vi "Parse U8 Ctl Regs.vi"(9 "NTeeths In":T6, 10 "FullyCustomTeeths In":T4, 11 "U8":T2[](array[typedef])) -> (1 "NTeeths Out":T6, 2 "FullyCustomTeeths In":T4)   [LabVIEW 2011, in "Engine Sim System Explorer.lvlib"]
uses:
  Engine Sim System Explorer.lvlib
  TypeDefs/NTeethRegs.ctl
  TypeDefs/FullyCustomRegs.ctl
  <userlib>/_FPGA Interface Advanced Tools/FPGA Bitfile Utility/TypeDefs/Scalar Register.ctl
  <userlib>/_FPGA Interface Advanced Tools/FPGA Bitfile Utility/FPGA Bitfile Utility.lvlib
panel:
  in  "FullyCustomTeeths Profile Names":T1(array[cluster])
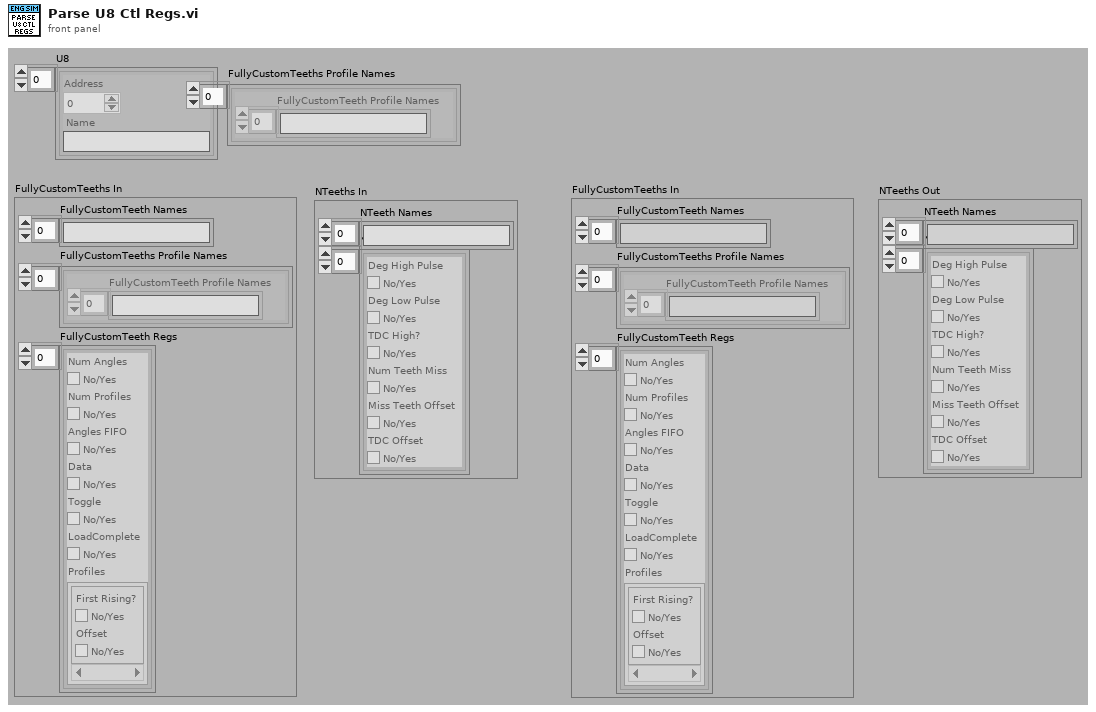
[diagram p1: front panel]
types:
  T1 = cluster{"FullyCustomTeeth Profile Names":string[]}[]
  T2 = typedef "FPGA Bitfile Utility.lvlib/Scalar Register.ctl" = cluster{"Address":u32, "Name":string}
  T3 = typedef "Engine Sim System Explorer.lvlib/FullyCustomRegs.ctl" = cluster{"Num Angles":bool, "Num Profiles":bool, "Angles FIFO":bool, "Data":bool, "Toggle":bool, "LoadComplete":bool, "Profiles":cluster{"First Rising?":bool, "Offset":bool}[]}
  T4 = cluster{"FullyCustomTeeth Names":string[], "FullyCustomTeeths Profile Names":cluster{"FullyCustomTeeth Profile Names":string[]}[], "FullyCustomTeeth Regs":T3[]}
  T5 = typedef "Engine Sim System Explorer.lvlib/NTeethRegs.ctl" = cluster{"Deg High Pulse":bool, "Deg Low Pulse":bool, "TDC High?":bool, "Num Teeth Miss":bool, "Miss Teeth Offset":bool, "TDC Offset":bool}
  T6 = cluster{"NTeeth Names":string[], "NTeeth Regs":T5[]}
  T7 = cluster{"FullyCustomTeeth Profile Names":string[]}
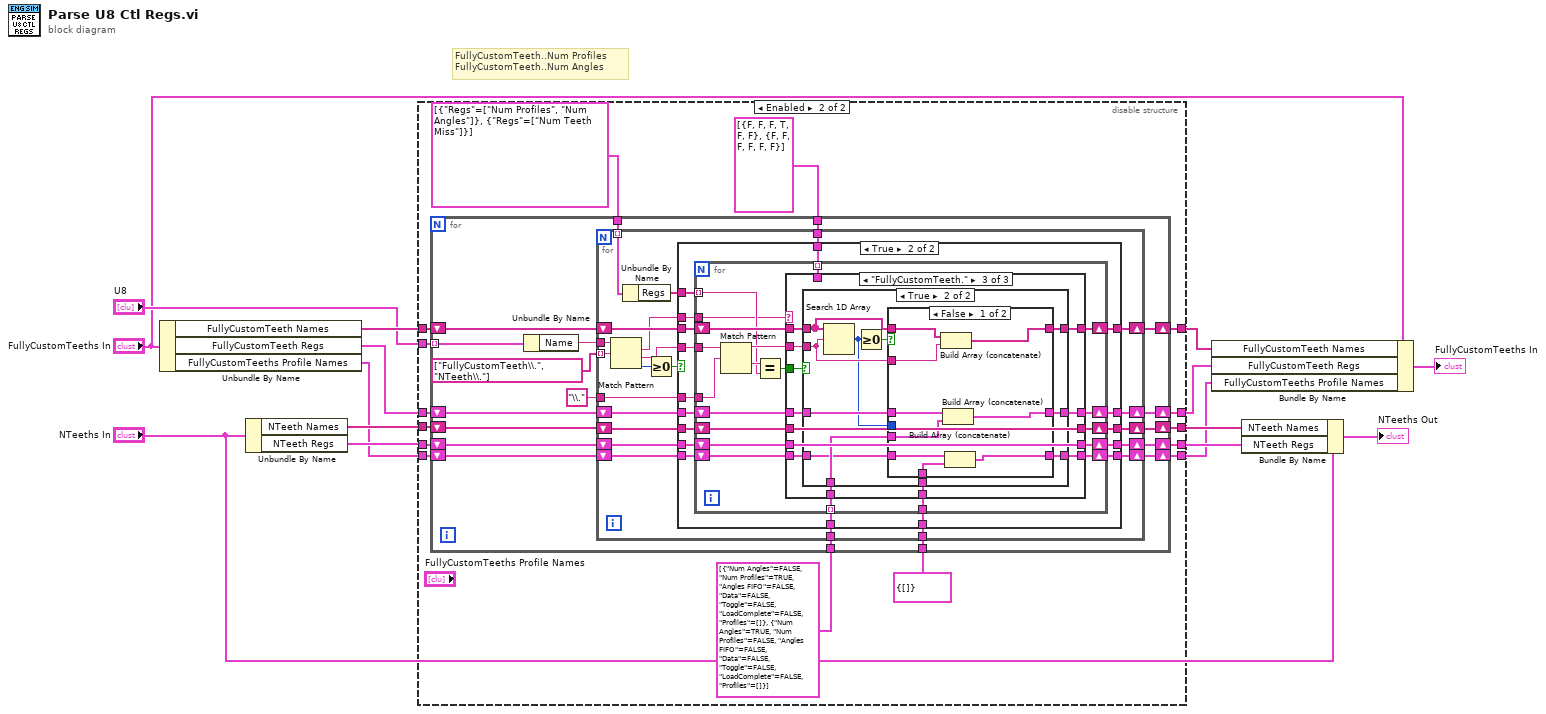
[diagram p0: block diagram]
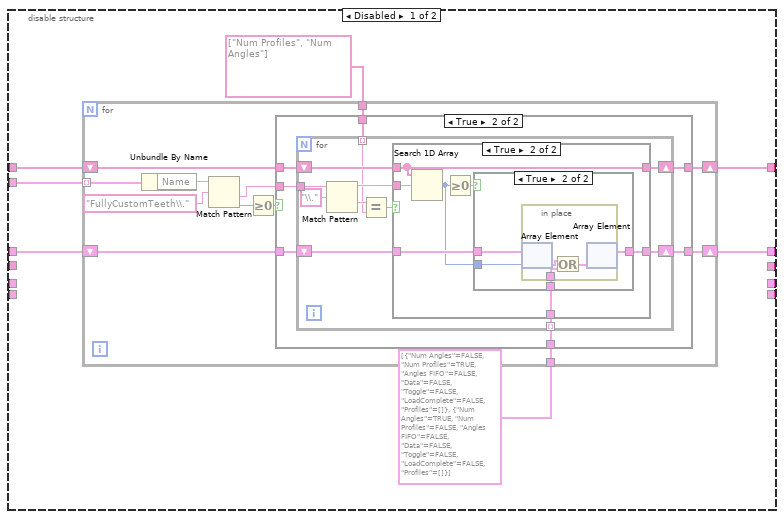
[diagram p2: hidden frame]
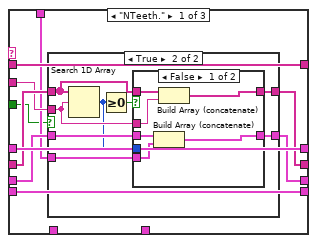
[diagram p7: hidden frame]
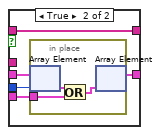
[diagram p9: hidden frame]
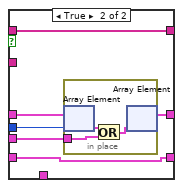
[diagram p12: hidden frame]
diagram:
  # "FullyCustomTeeth..Num Profiles\nFullyCustomTeeth..Num Angles"
  n1 = Unbundle By Name("FullyCustomTeeths In") -> ("FullyCustomTeeth Names"=w6:string[], "FullyCustomTeeth Regs"=w7:T3[], "FullyCustomTeeths Profile Names"=w2:T1)
  n2 = Unbundle By Name("NTeeths In") -> ("NTeeth Names"=w8:string[], "NTeeth Regs"=w9:T5[])
  n3 = disable-structure shown="Enabled" {
    disable-tunnel: w6 -> [w22 w85]
    disable-tunnel: w7 -> [w21 w84]
    disable-tunnel: "U8" -> [w20 w86]
    disable-tunnel: [w17 w83] -> w11
    disable-tunnel: [w16 w82] -> w10
    disable-tunnel: w9 -> [_ w79]
    disable-tunnel: w8 -> [_ w78]
    disable-tunnel: [_ w77] -> w14
    disable-tunnel: [_ w76] -> w15
    disable-tunnel: w2 -> [_ w75]
    disable-tunnel: [_ w73] -> w1
    frame Disabled {
      n4 = for {
        tunnel: w20 -> [w34] mode=indexing
        tunnel: T3[] [{"Num Angles"=FALSE, "Num Profiles"=TRUE, "Angles FIFO"=FALSE, "Data"=FALSE, "Toggle"=FALSE, "LoadComplete"=FALSE, "Profiles"=[]}, {"Num Angles"=TRUE, "Num Profiles"=FALSE, "Angles FIFO"=FALSE, "Data"=FALSE, "Toggle"=FALSE, "LoadComplete"=FALSE, "Profiles"=[]}] -> [w28]
        shift-right: [w27] -> w17
        shift-left: w21 -> [w26]
        shift-right: [w25] -> w16
        shift-left: w22 -> [w24]
        tunnel: string[] ["Num Profiles", "Num Angles"] ("Regs") -> [w23]
        n5 = Unbundle By Name(w34) -> ("Name"=w33:string)
        n6 = Match Pattern(string=w33, regular expression="FullyCustomTeeth\\.") -> (after substring=w29:string, offset past match=w31:i32)  [unwired: 1 in, 2 out]
        n7 = Greater Or Equal To 0?(x=w31) -> (x >= 0?=w30:bool)
        n8 = case shown="True" w30 {
          tunnel: w29 -> [_ w43]
          tunnel: w28 -> [_ w42]
          tunnel: [w35 w41] -> w27
          tunnel: w26 -> [w35 w40]
          tunnel: [w36 w39] -> w25
          tunnel: w24 -> [w36 w38]
          tunnel: w23 -> [_ w37]
          frame False {
          }
          frame True {
            n9 = for {
              tunnel: w43 -> [w54]
              tunnel: w42 -> [w49] mode=indexing
              tunnel: w37 -> [w44] mode=indexing
              shift-right: [w46] -> w39
              shift-left: w38 -> [w45]
              shift-right: [w48] -> w41
              shift-left: w40 -> [w47]
              n10 = Match Pattern(string=w54, regular expression="\\.") -> (before substring=w50:string, after substring=w52:string)  [unwired: 1 in, 2 out]
              n11 = Equal?(x=w52, y=w44) -> (x = y?=w51:bool)
              n12 = case shown="True" w51 {
                tunnel: w50 -> [_ w63]
                tunnel: w49 -> [_ w59]
                tunnel: [w55 w58] -> w48
                tunnel: w47 -> [w55 w60]
                tunnel: [w56 w62] -> w46
                tunnel: w45 -> [w56 w62]
                frame False {
                }
                frame True {
                  n13 = Search 1D Array(1D array=w62, element=w63) -> (index of element=w57:i32)  [unwired: 1 in]
                  n14 = Greater Or Equal To 0?(x=w57) -> (x >= 0?=w61:bool)
                  n15 = case shown="True" w61 {
                    tunnel: w60 -> [w64 w68]
                    tunnel: w59 -> [_ w67]
                    tunnel: [w64 w66] -> w58
                    tunnel: w57 -> [_ w65]
                    frame False {
                    }
                    frame True {
                      n16 = in-place {
                        in-place-border: w67 -> [w70]
                        n17 = in-place-array #1(w68, w65) -> (w71:T3)
                        n18 = Or(x=w71, y=w70) -> (x .or. y?=w69:T3)
                        n19 = in-place-array #1(w69) -> (w66:T3[])  [unwired: 1 out]
                      }
                    }
                  }
                }
              }
            }
          }
        }
      }
    }
    frame Enabled {
      n20 = for {
        tunnel: w86 -> [w104] mode=indexing
        tunnel: T3[] [{"Num Angles"=FALSE, "Num Profiles"=TRUE, "Angles FIFO"=FALSE, "Data"=FALSE, "Toggle"=FALSE, "LoadComplete"=FALSE, "Profiles"=[]}, {"Num Angles"=TRUE, "Num Profiles"=FALSE, "Angles FIFO"=FALSE, "Data"=FALSE, "Toggle"=FALSE, "LoadComplete"=FALSE, "Profiles"=[]}] -> [w102]
        shift-right: [w101] -> w83
        shift-left: w84 -> [w100]
        shift-right: [w99] -> w82
        shift-left: w85 -> [w98]
        tunnel: cluster{"Regs":string[]}[] [{"Regs"=["Num Profiles", "Num Angles"]}, {"Regs"=["Num Teeth Miss"]}] -> [w96]
        shift-right: [w95] -> w76
        shift-left: w79 -> [w94]
        tunnel: T5[] [{"Deg High Pulse"=FALSE, "Deg Low Pulse"=FALSE, "TDC High?"=FALSE, "Num Teeth Miss"=TRUE, "Miss Teeth Offset"=FALSE, "TDC Offset"=FALSE}, {"Deg High Pulse"=FALSE, "Deg Low Pulse"=FALSE, "TDC High?"=FALSE, "Num Teeth Miss"=FALSE, "Miss Teeth Offset"=FALSE, "TDC Offset"=FALSE}] -> [w93]
        shift-right: [w91] -> w77
        shift-left: w78 -> [w90]
        shift-right: [w88] -> w73
        shift-left: w75 -> [w89]
        tunnel: T7 {"FullyCustomTeeth Profile Names"=[]} ("FullyCustomTeeth") -> [w87]
        n21 = Unbundle By Name(w104) -> ("Name"=w103:string)
        n22 = for {
          tunnel: w103 -> [w126]
          tunnel: w102 -> [w122]
          tunnel: string[] ["FullyCustomTeeth\\.", "NTeeth\\."] -> [w117] mode=indexing
          shift-right: [w119] -> w99
          shift-left: w98 -> [w118]
          shift-right: [w121] -> w101
          shift-left: w100 -> [w120]
          tunnel: w96 -> [w116] mode=indexing
          shift-right: [w113] -> w95
          shift-left: w94 -> [w112]
          tunnel: w93 -> [w111]
          tunnel: "\\." ("regular expression") -> [w110]
          shift-right: [w109] -> w91
          shift-left: w90 -> [w108]
          shift-right: [w106] -> w88
          shift-left: w89 -> [w107]
          tunnel: w87 -> [w105]
          n23 = Match Pattern(string=w126, regular expression=w117) -> (match substring=w114:string, after substring=w123:string, offset past match=w125:i32)  [unwired: 1 in, 1 out]
          n24 = Unbundle By Name(w116) -> ("Regs"=w115:string[])
          n25 = Greater Or Equal To 0?(x=w125) -> (x >= 0?=w124:bool)
          n26 = case shown="True" w124 {
            tunnel: w123 -> [_ w148]
            tunnel: w122 -> [_ w147]
            tunnel: [w130 w146] -> w121
            tunnel: w120 -> [w130 w145]
            tunnel: [w131 w144] -> w119
            tunnel: w118 -> [w131 w143]
            tunnel: w115 -> [_ w142]
            tunnel: w114 -> [_ w141]
            tunnel: [w129 w140] -> w113
            tunnel: w112 -> [w129 w139]
            tunnel: w111 -> [_ w138]
            tunnel: w110 -> [_ w137]
            tunnel: [w128 w136] -> w109
            tunnel: w108 -> [w128 w135]
            tunnel: w107 -> [w127 w134]
            tunnel: [w127 w133] -> w106
            tunnel: w105 -> [_ w132]
            frame False {
            }
            frame True {
              n27 = for {
                tunnel: w148 -> [w168]
                tunnel: w147 -> [w164] mode=indexing
                shift-right: [w161] -> w144
                shift-left: w143 -> [w160]
                shift-right: [w163] -> w146
                shift-left: w145 -> [w162]
                tunnel: w142 -> [w159] mode=indexing
                tunnel: w141 -> [w158]
                shift-right: [w157] -> w140
                shift-left: w139 -> [w154]
                tunnel: w138 -> [w156] mode=indexing
                tunnel: w137 -> [w155]
                shift-right: [w153] -> w136
                shift-left: w135 -> [w152]
                shift-right: [w150] -> w133
                shift-left: w134 -> [w151]
                tunnel: w132 -> [w149]
                n28 = Match Pattern(string=w168, regular expression=w155) -> (before substring=w165:string, after substring=w167:string)  [unwired: 1 in, 2 out]
                n29 = Equal?(x=w167, y=w159) -> (x = y?=w166:bool)
                n30 = case shown="\"FullyCustomTeeth.\"" w158 {
                  tunnel: w166 -> [w170 _ w219]
                  tunnel: w165 -> [w173 _ w218]
                  tunnel: w164 -> [_ _ w217]
                  tunnel: [w177 w206 w216] -> w163
                  tunnel: w162 -> [w177 w206 w215]
                  tunnel: [w178 w207 w214] -> w161
                  tunnel: w160 -> [w178 w207 w213]
                  tunnel: [w174 w205 w212] -> w157
                  tunnel: w156 -> [w171 _ _]
                  tunnel: w154 -> [w172 w205 w212]
                  tunnel: [w175 w204 w211] -> w153
                  tunnel: w152 -> [w176 w204 w211]
                  tunnel: w151 -> [w169 w203 w210]
                  tunnel: [w169 w203 w209] -> w150
                  tunnel: w149 -> [_ _ w208]
                  frame "NTeeth." {
                    n31 = case shown="True" w170 {
                      tunnel: w173 -> [_ w184]
                      tunnel: [w179 w186] -> w174
                      tunnel: w172 -> [w179 w187]
                      tunnel: [w180 w183] -> w175
                      tunnel: w176 -> [w180 w185]
                      tunnel: w171 -> [_ w181]
                      frame False {
                      }
                      frame True {
                        n32 = Search 1D Array(1D array=w185, element=w184) -> (index of element=w182:i32)  [unwired: 1 in]
                        n33 = Greater Or Equal To 0?(x=w182) -> (x >= 0?=w188:bool)
                        n34 = case shown="False" w188 {
                          tunnel: w187 -> [w194 w198]
                          tunnel: w181 -> [w193 w196]
                          tunnel: [w192 w195] -> w186
                          tunnel: w185 -> [w191 w199]
                          tunnel: w184 -> [w190 _]
                          tunnel: [w189 w199] -> w183
                          tunnel: w182 -> [_ w197]
                          frame False {
                            n35 = Build Array (concatenate)(w194, w193) -> (w192:T5[])
                            n36 = Build Array (concatenate)(w191, w190) -> (w189:string[])
                          }
                          frame True {
                            n37 = in-place {
                              in-place-border: w196 -> [w201]
                              n38 = in-place-array #2(w198, w197) -> (w202:T5)
                              n39 = Or(x=w202, y=w201) -> (x .or. y?=w200:T5)
                              n40 = in-place-array #2(w200) -> (w195:T5[])  [unwired: 1 out]
                            }
                          }
                        }
                      }
                    }
                  }
                  frame Default {
                  }
                  frame "FullyCustomTeeth." {
                    n41 = case shown="True" w219 {
                      tunnel: w218 -> [_ w229]
                      tunnel: w217 -> [_ w232]
                      tunnel: [w221 w231] -> w216
                      tunnel: w215 -> [w221 w233]
                      tunnel: [w222 w228] -> w214
                      tunnel: w213 -> [w222 w230]
                      tunnel: w210 -> [w220 w226]
                      tunnel: [w220 w225] -> w209
                      tunnel: w208 -> [_ w224]
                      frame False {
                      }
                      frame True {
                        n42 = Search 1D Array(1D array=w230, element=w229) -> (index of element=w227:i32)  [unwired: 1 in]
                        n43 = Greater Or Equal To 0?(x=w227) -> (x >= 0?=w223:bool)
                        n44 = case shown="False" w223 {
                          tunnel: w233 -> [w242 w247]
                          tunnel: w232 -> [w241 w245]
                          tunnel: [w240 w244] -> w231
                          tunnel: w230 -> [w239 w248]
                          tunnel: w229 -> [w238 _]
                          tunnel: [w237 w248] -> w228
                          tunnel: w227 -> [_ w246]
                          tunnel: w226 -> [w236 w243]
                          tunnel: [w235 w243] -> w225
                          tunnel: w224 -> [w234 _]
                          frame False {
                            n45 = Build Array (concatenate)(w239, w238) -> (w237:string[])
                            n46 = Build Array (concatenate)(w242, w241) -> (w240:T3[])
                            n47 = Build Array (concatenate)(w236, w234) -> (w235:T1)
                          }
                          frame True {
                            n48 = in-place {
                              in-place-border: w245 -> [w250]
                              n49 = in-place-array #3(w247, w246) -> (w251:T3)
                              n50 = Or(x=w251, y=w250) -> (x .or. y?=w249:T3)
                              n51 = in-place-array #3(w249) -> (w244:T3[])  [unwired: 1 out]
                            }
                          }
                        }
                      }
                    }
                  }
                }
              }
            }
          }
        }
      }
    }
  }
  n52 = Bundle By Name(cluster="FullyCustomTeeths In", "FullyCustomTeeth Names"=w10, "FullyCustomTeeth Regs"=w11, "FullyCustomTeeths Profile Names"=w1) -> (→"FullyCustomTeeths In":T4)
  n53 = Bundle By Name(cluster="NTeeths In", "NTeeth Names"=w14, "NTeeth Regs"=w15) -> (→"NTeeths Out":T6)
